vi "Actor Event.vi"(8 "Queue Mailbox":refnum<data-value>, 9 "Self Alias":string, 10 "Queue of Event Self":refnum<queue>, 11 "Event jettl":refnum<class "Event jettl.lvclass">) -> ()   [LabVIEW 2021, in "jettl.lvlib" / "Base Event jettl.lvlib" / "Base Event jettl.lvclass"]
uses:
  Base Event jettl.lvclass
  Base Event jettl.lvclass/Base Event jettl.ctl
  Self Event/Self Event.lvlib
  Event jettl/Event jettl.lvclass
  jettl.lvlib
  jettl Msg Last Ack Event/jettl Msg Last Ack Event.lvlib
  C:/git/jettl/src/jettl/jettl/jettl.lvclass
  C:/git/jettl/src/jettl Msg Merge Error/Merge Error/Merge Error.lvclass
  C:/git/jettl/src/jettl/Event jettl/Event jettl.lvclass
  C:/git/jettl/src/jettl Msg Override Error/Override Error/Override Error.lvclass
  C:/git/jettl/src/jettl Msg Setup/Setup/Setup.lvclass
  C:/git/jettl/src/jettl Msg Teardown/Teardown/Teardown.lvclass
  C:/git/jettl/src/jettl/Base Event jettl/Base Event jettl/Base Event jettl.lvclass
  jettl Msg Last Ack Event/Last Ack Event Msg Strategy/Last Ack Event Msg Strategy.lvclass
  C:/git/jettl/src/jettl/jettl Msg Last Ack Event/Event Last Ack Msg Strategy/Last Ack Event Msg Strategy.lvclass
  C:/git/jettl/src/jettl/Msg Strategy/Msg Strategy.lvclass
  Msg Strategy/Msg Strategy.lvclass
  Queue Mailbox/Queue Mailbox/Queue Mailbox.lvclass
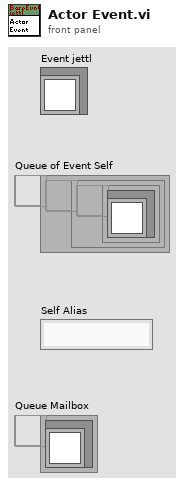
[diagram p1: front panel]
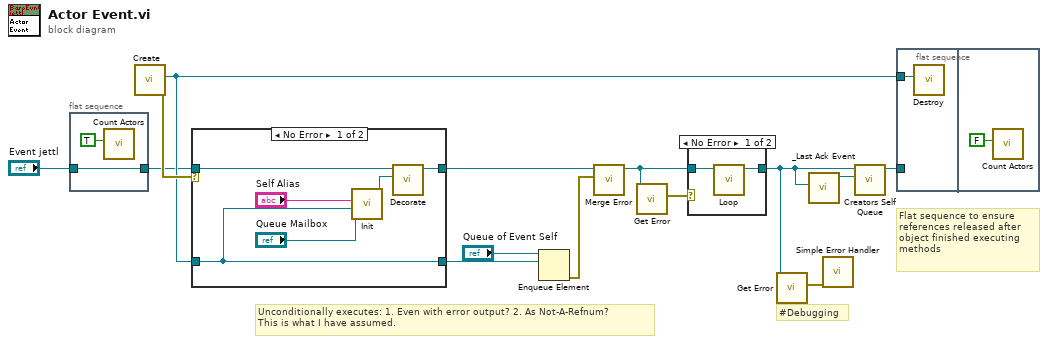
[diagram p0: block diagram]
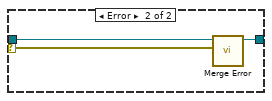
[diagram p2: hidden frame]
diagram:
  # "Flat sequence to ensure references released after object finished executing methods"
  # "#Debugging"
  # "Unconditionally executes: 1. Even with error output? 2. As Not-A-Refnum?\nThis is what I have assumed."
  n1 = flat-sequence {
    tunnel: [w15] -> w6
    tunnel: "Event jettl" -> [w15]
    frame #0 {
      n2 = call "Count Actors.vi"("Increment?"=TRUE) -> ()  [unwired: 11 in]
    }
  }
  n3 = call "Create.vi"() -> ("error out"=w9:errorcluster, "Self Event"=w8:refnum<data-value>)  [unwired: 10 in]
  n4 = case shown="No Error" w9 {
    selector: w9 -> [_ w24]
    tunnel: [w20 w25] -> w12
    tunnel: w6 -> [w22 w23]
    tunnel: w8 -> [w17 _]
    tunnel: [w17 _] -> w11
    frame No Error {
      n5 = call "Init.vi"("Queue Mailbox"="Queue Mailbox", "Self"=w17, "Self Alias"="Self Alias") -> ("Base Event jettl out"=w21:refnum<class "Base Event jettl.lvclass">)  [unwired: 8 in]
      n6 = call-dynamic "Decorate.vi"("Event jettl"=w21, "Event jettl in"=w22) -> ("Event jettl out"=w20:refnum<class "Event jettl.lvclass">)  [unwired: 9 in]
    }
    frame Error {
      n7 = call-dynamic "Merge Error.vi"("Error"=w24, "Merge Error in"=w23) -> ("Merge Error out"=w25:refnum<class "Event jettl.lvclass">)  [unwired: 9 in]
    }
  }
  n8 = Enqueue Element(queue="Queue of Event Self", element=w11) -> (error out=w13:errorcluster)  [unwired: 2 in, 2 out]
  n9 = call-dynamic "Merge Error.vi"("Error"=w13, "Merge Error in"=w12) -> ("Merge Error out"=w14:refnum<class "Event jettl.lvclass">)  [unwired: 9 in]
  n10 = call-dynamic "Get Error.vi"("jettl in"=w14) -> ("Error"=w10:errorcluster)  [unwired: 10 in]
  n11 = case shown="No Error" w10 {
    tunnel: w14 -> [w27 w28]
    tunnel: [w26 w28] -> w3
    frame No Error {
      n12 = call-dynamic "Loop.vi"("Event jettl in"=w27) -> ("Event jettl out"=w26:refnum<class "Event jettl.lvclass">)  [unwired: 10 in]
    }
    frame Error {
    }
  }
  n13 = call-dynamic "Get Error.vi"("jettl in"=w3) -> ("Error"=w4:errorcluster)  [unwired: 10 in]
  n14 = call "_Last Ack Event.vi"("Event jettl"=w3) -> ("Event Last Ack Msg Strategy out"=w1:refnum<class "Last Ack Event Msg Strategy.lvclass">)  [unwired: 10 in]
  n15 = call <vilib>:"Simple Error Handler.vi"("error in (no error)"=w4) -> ()  [unwired: 4 in, 5 out]
  n16 = call-dynamic "Creators Self Queue.vi"("Msg Strategy"=w1, "Event jettl in"=w3) -> ("Event jettl out"=w2:refnum<class "Event jettl.lvclass">)  [unwired: 9 in]
  n17 = flat-sequence {
    tunnel: w8 -> [w29]
    tunnel: w2 -> [_]
    frame #0 {
      n18 = call "Destroy.vi"("Self Event"=w29) -> ()  [unwired: 10 in, 1 out]
    }
    frame #1 {
      n19 = call "Count Actors.vi"("Increment?"=FALSE) -> ()  [unwired: 11 in]
    }
  }
